vi "initialise.vi"(8 "error in (no error)":errorcluster, 11 "GenericPlugin in":refnum<class "StageMH110930Scientifica.lvclass">) -> (0 "error out":errorcluster, 3 "GenericPlugin out":refnum<class "StageMH110930Scientifica.lvclass">)   [LabVIEW 2010, in "StageMH110930Scientifica.lvclass"]
doc: "The dynamic dispatch-version of this VI initalises the plug-in object by allocating and initalising any dynamic resources need."
uses:
  StageMH110930Scientifica.lvclass
  StageDL090409Scaffold/StageDL090409Scaffold/StageDL090409Scaffold.lvclass
  <vilib>/Instr/_visa.llb/VISA Configure Serial Port (Instr).vi
  common/classes/ErrorController/ErrorController/class_data.vi
  common/classes/ErrorController/ErrorController/ErrorController.lvclass
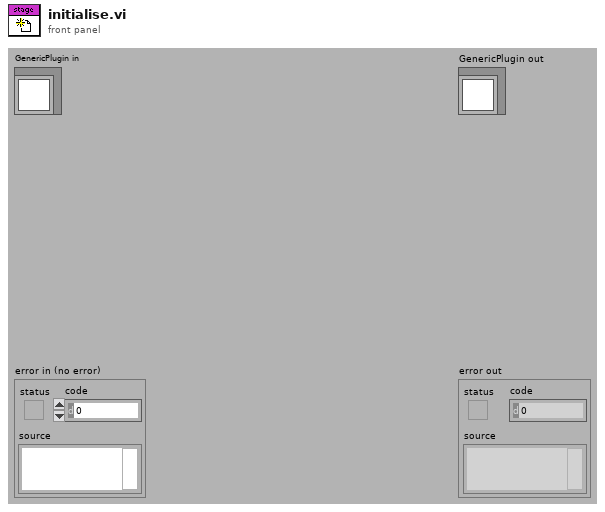
[diagram p1: front panel]
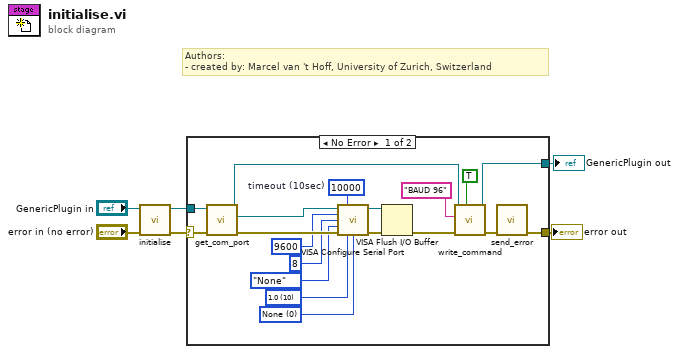
[diagram p0: block diagram]
diagram:
  # "Authors: \n- created by: Marcel van 't Hoff, University of Zurich, Switzerland"
  n1 = call-parent "initialise.vi"("error in (no error)"="error in (no error)", "GenericPlugin in"="GenericPlugin in") -> ("error out"=w4:errorcluster, "GenericPlugin out"=w1:refnum<class "StageMH110930Scientifica.lvclass">)  [unwired: 8 in]
  n2 = case shown="No Error" w4 {
    selector: w4 -> [w23 w27]
    tunnel: [w11 w27] -> w3
    tunnel: [w14 w26] -> w2
    tunnel: w1 -> [w25 w26]
    frame No Error {
      w16 = u16 0 items=["None", "XON/XOFF", "RTS/CTS", "XON/XOFF & RTS/CTS", "DTR/DSR", "XON/XOFF & DTR/DSR"] ("flow control (0:none)")
      w17 = u16 10 items=["1.0"=10, "1.5"=15, "2.0"=20] ("stop bits (10: 1 bit)")
      w21 = u32 10000  # timeout (10sec)
      n3 = call-dynamic "get_com_port.vi"("error in (no error)"=w23, "StageMH110930Scientifica in"=w25) -> ("error out"=w22:errorcluster, "serial port name"=w24:refnum<visa-resource-name>, "StageMH110930Scientifica out"=w15:refnum<class "StageMH110930Scientifica.lvclass">)  [unwired: 7 in]
      n4 = call-poly "VISA Configure Serial Port"("VISA resource name"=w24, "timeout (10sec)"=w21, "baud rate (9600)"=u32 9600, "data bits (8)"=u16 8, "parity (0:none)"=enum16{"None", "Odd", "Even", "Mark", "Space"}."None", "error in (no error)"=w22, "stop bits (10: 1 bit)"=w17, "flow control (0:none)"=w16) -> ("VISA resource name out"=w9:refnum<visa-resource-name>, "error out"=w8:errorcluster)  [unwired: 6 in]
      n5 = VISA Flush I/O Buffer(VISA resource name=w9, error in (no error)=w8) -> (error out=w7:errorcluster)  [unwired: 1 in, 1 out]
      n6 = call-dynamic "write_command.vi"("read (T)"=TRUE, "error in (no error)"=w7, "string to write"="BAUD 96", "StageMH110930Scientifica in"=w15) -> ("error out"=w12:errorcluster, "StageMH110930Scientifica out"=w14:refnum<class "StageMH110930Scientifica.lvclass">)  [unwired: 4 in, 2 out]
      n7 = call "send_error.vi"("error in (no error)"=w12) -> ("error out"=w11:errorcluster)  [unwired: 10 in]
    }
    frame Error {
    }
  }
  "error out" <- w3
  "GenericPlugin out" <- w2
